vi "Path as Path (UTF-8 Path).vi"(10 "Path":refnum<class "UTF-8 Path.lvclass">) -> (2 "Path":path)   [LabVIEW 2020, in "G-Unicode.lvlib"]
doc: "Converts the input path to a raw UTF-8 encoded LabVIEW path. Valid inputs are a UTF-8 Path class or LabVIEW path."
uses:
  G-Unicode.lvlib
  Types/UTF-8 Path/UTF-8 Path.lvclass
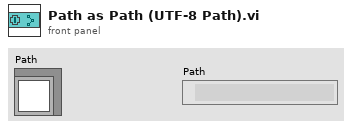
[diagram p1: front panel]
types:
  T1 = typedef "G-Unicode.lvlib/Encoded UTF-8 Path.ctl" = path
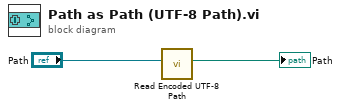
[diagram p0: block diagram]
diagram:
  n1 = call "Read Encoded UTF-8 Path.vi"("UTF-8 Path"="Path") -> ("Encoded UTF-8 Path"=→"Path":T1)  [unwired: 10 in]
